vi "NI-IIR Filter with I.C. PtByPt.vi"(6 "Initial Y Conditions":dbl[](array[numeric]), 7 "initialize":bool, 8 "Initial X Conditions":dbl[](array[numeric]), 9 "Forward Coefficients":dbl[](array[numeric]), 10 "Reverse Coefficients":dbl[](array[numeric]), 11 "x":dbl format="%0.2f") -> (0 "Final X Conditions":dbl[](array[numeric]), 1 "error":i32, 3 "Filtered x":dbl format="%0.2f", 4 "Final Y Conditions":dbl[](array[numeric]))   [LabVIEW 2020]
doc: "Filters <B>x</B> using the IIR filter specified by <B>Reverse Coefficients</B> and <B>Forward Coefficients</B>."
uses:
  <vilib>/Analysis/3filter.llb/IIR Filter with I.C. (DBL).vi
  <vilib>/Analysis/NI_AALBase.lvlib
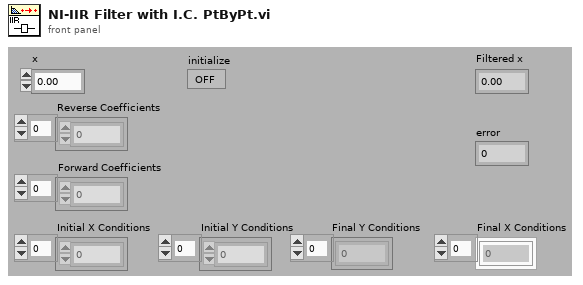
[diagram p1: front panel]
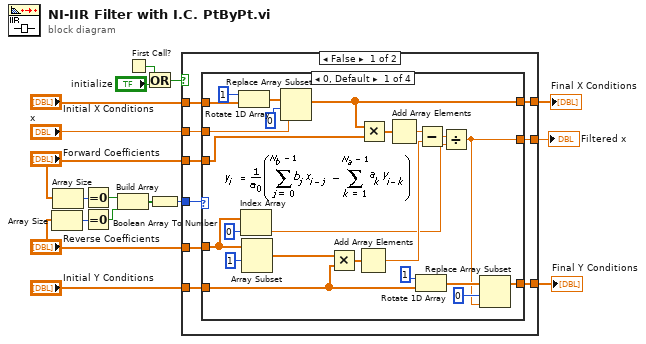
[diagram p0: block diagram]
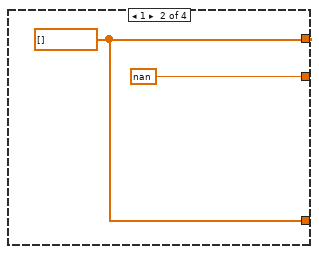
[diagram p2: hidden frame]
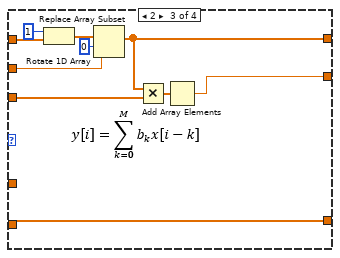
[diagram p3: hidden frame]
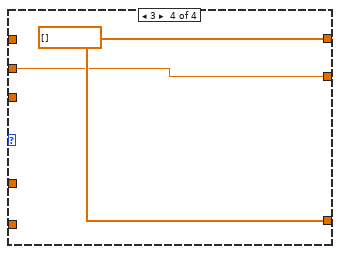
[diagram p4: hidden frame]
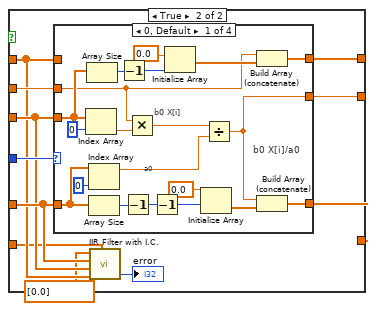
[diagram p5: hidden frame]
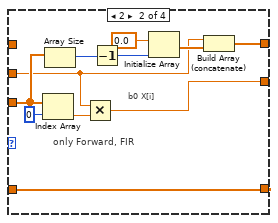
[diagram p6: hidden frame]
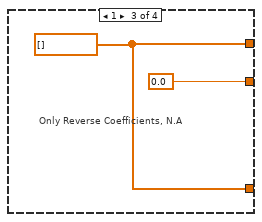
[diagram p7: hidden frame]
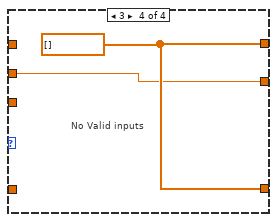
[diagram p8: hidden frame]
diagram:
  n1 = Array Size(array="Reverse Coefficients") -> (size(s)=w9:i32)
  n2 = Array Size(array="Forward Coefficients") -> (size(s)=w8:i32)
  n3 = Equal To 0?(x=w8) -> (x = 0?=w10:bool)
  n4 = Equal To 0?(x=w9) -> (x = 0?=w11:bool)
  n5 = Build Array(w10, w11) -> (w7:bool[])
  n6 = First Call?() -> (First Call?: T/F=w3:bool)
  n7 = Or(x=w3, y="initialize") -> (x .or. y?=w1:bool)
  n8 = Boolean Array To Number(Boolean array=w7) -> (number=w4:u32)
  n9 = case shown="False" w1 {
    tunnel: "Reverse Coefficients" -> [w26 w69]
    tunnel: "Forward Coefficients" -> [w25 w68]
    tunnel: "Initial X Conditions" -> [w24 w67]
    tunnel: "Initial Y Conditions" -> [w23 w66]
    tunnel: [w19 w74] -> w16
    tunnel: [w22 w72] -> w13
    tunnel: [w21 w73] -> w12
    tunnel: "x" -> [w20 w71]
    tunnel: w4 -> [w18 w70]
    frame False {
      n10 = case shown="0, Default" w18 {
        tunnel: w24 -> [w37 _ w57 _]
        tunnel: w26 -> [w29 _ _ _]
        tunnel: w23 -> [w45 _ w52 _]
        tunnel: w25 -> [w35 _ w55 _]
        tunnel: [w36 w51 w53 w63] -> w22
        tunnel: [w41 w51 w52 w63] -> w21
        tunnel: w20 -> [w34 _ w56 w62]
        tunnel: [w31 nan ("Input_X") w54 w62] -> w19
        frame 0, Default {
          n11 = Rotate 1D Array(1:w37, 2:i16 1 ("n")) -> (0:w39:dbl[])
          n12 = Index Array(array=w29, index=0 ("Index")) -> (element=w27:dbl)
          n13 = Array Subset(array=w29, index=1 ("Array Index")) -> (w33:dbl[])  [unwired: 1 in]
          n14 = Replace Array Subset(array=w39, new element=w34, index=0 ("Index")) -> (w36:dbl[])
          n15 = Multiply(x=w33, y=w45) -> (x*y=w48:dbl[])
          n16 = Add Array Elements(numeric array=w48) -> (sum=w46:dbl)
          n17 = Multiply(x=w36, y=w35) -> (x*y=w49:dbl[])
          n18 = Add Array Elements(numeric array=w49) -> (sum=w47:dbl)
          n19 = Rotate 1D Array(1:w45, 2:i16 1 ("n")) -> (0:w43:dbl[])
          n20 = Subtract(x=w47, y=w46) -> (x-y=w30:dbl)
          n21 = Divide(x=w30, y=w27) -> (x/y=w31:dbl)
          n22 = Replace Array Subset(array=w43, new element=w31, index=0 ("Index")) -> (w41:dbl[])
        }
        frame 1 {
          w51 = dbl[] []
        }
        frame 2 {
          n23 = Rotate 1D Array(1:w57, 2:i16 1 ("n")) -> (0:w59:dbl[])
          n24 = Replace Array Subset(array=w59, new element=w56, index=0 ("Index")) -> (w53:dbl[])
          n25 = Multiply(x=w53, y=w55) -> (x*y=w61:dbl[])
          n26 = Add Array Elements(numeric array=w61) -> (sum=w54:dbl)
        }
        frame 3 {
          w63 = dbl[] []
        }
      }
    }
    frame True {
      n27 = case shown="0, Default" w70 {
        tunnel: w67 -> [_ _ _ _]
        tunnel: w68 -> [w86 w100 _ _]
        tunnel: [w79 w96 0.0 w108] -> w74
        tunnel: [w83 w97 w107 w109] -> w72
        tunnel: [w82 w95 w107 w109] -> w73
        tunnel: w71 -> [w84 w98 _ w108]
        tunnel: w69 -> [w75 w95 _ _]
        frame 0, Default {
          # "b0 X[i]/a0"
          # "a0"
          # "b0 X[i]"
          n28 = Index Array(array=w86, index=0 ("Index")) -> (element=w90:dbl)
          n29 = Array Size(array=w86) -> (size(s)=w94:i32)
          n30 = Index Array(array=w75, index=0 ("Index")) -> (element=w76:dbl)
          n31 = Array Size(array=w75) -> (size(s)=w89:i32)
          n32 = Decrement(x=w94) -> (x-1=w93:i32)
          n33 = Decrement(x=w89) -> (x-1=w80:i32)
          n34 = Multiply(x=w84, y=w90) -> (x*y=w78:dbl)
          n35 = Decrement(x=w80) -> (x-1=w88:i32)
          n36 = Initialize Array(0.0 ("Element Data"), w93) -> (w85:dbl[])
          n37 = Initialize Array(0.0 ("Element Data"), w88) -> (w81:dbl[])
          n38 = Divide(x=w78, y=w76) -> (x/y=w79:dbl)
          n39 = Build Array (concatenate)(w84, w85) -> (w83:dbl[])
          n40 = Build Array (concatenate)(w79, w81) -> (w82:dbl[])
        }
        frame 2 {
          # "b0 X[i]"
          # "only Forward, FIR"
          n41 = Index Array(array=w100, index=0 ("Index")) -> (element=w101:dbl)
          n42 = Array Size(array=w100) -> (size(s)=w105:i32)
          n43 = Multiply(x=w98, y=w101) -> (x*y=w96:dbl)
          n44 = Decrement(x=w105) -> (x-1=w104:i32)
          n45 = Initialize Array(0.0 ("Element Data"), w104) -> (w99:dbl[])
          n46 = Build Array (concatenate)(w98, w99) -> (w97:dbl[])
        }
        frame 1 {
          w107 = dbl[] []
          # "Only Reverse Coefficients, N.A"
        }
        frame 3 {
          w109 = dbl[] []
          # "No Valid inputs"
        }
      }
      n47 = call-poly <vilib>:"IIR Filter with I.C..vi"("Initial Y Conditions"=w66, "Initial X Conditions"=w67, "Forward Coefficients"=w68, "Reverse Coefficients"=w69, "X"=dbl[] [0.0]) -> ("error"=→"error":i32)  [unwired: 2 in, 3 out]
    }
  }
  "Filtered x" <- w16
  "Final X Conditions" <- w13
  "Final Y Conditions" <- w12
